vi "LVClass_WavefrontCorrectorSet Reset WavefrontCorrectorParameter to DefaultValue.vi"(0 "WavefrontCorrectorSet in":refnum<class "WavefrontCorrectorSet.lvclass">, 11 "error in (no error)":errorcluster) -> (4 "WavefrontCorrectorSet out":refnum<class "WavefrontCorrectorSet.lvclass">, 15 "error out":errorcluster)   [LabVIEW 2020, in "WavefrontCorrectorSet.lvclass"]
doc: "WavefrontCorrector parameter default value getter for parameter of type\nboolean.\n\n--------------------------------------------------------------------------------\n\n<B>wavefrontcorrector_setIn </B> : WavefrontCorrectorSet object.\n<B>wavefrontcorrector_setOut </B> : WavefrontCorrectorSet object.\n<B>parameter_name </B> : Parameter name.\n<B>default_value </B> : Parameter default value.\n<B>ErrorIn </B> : Error\n<B>ErrorOut </B> : Error\n\n--------------------------------------------------------------------------------"
uses:
  WavefrontCorrectorSet.lvclass
  WavefrontCorrectorSet.lvclass/WavefrontCorrectorSet.ctl
panel:
  in  "ListOfParametersToResetDefault":string[](array[string])
  in  "ResetAllParametersToDefault":bool
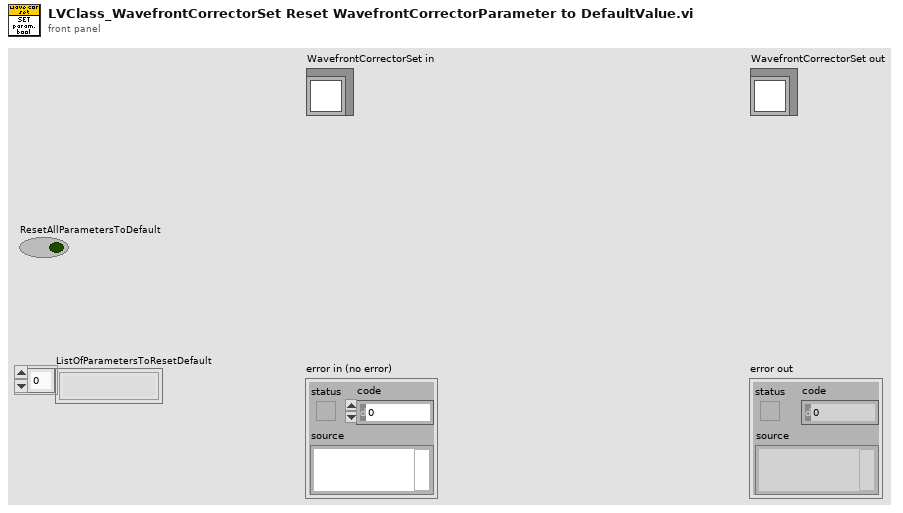
[diagram p1: front panel]
types:
  T1 = typedef "CameraParametersSetup.ctl" = cluster{"Name":string, "Type":T2, "Value":dbl, "BooleanValue":bool, "StringValue":string, "ConnectionParameter":bool}
  T2 = typedef "CameraParameters_Type.ctl" = enum16{"Integer", "Real", "String", "Boolean"}
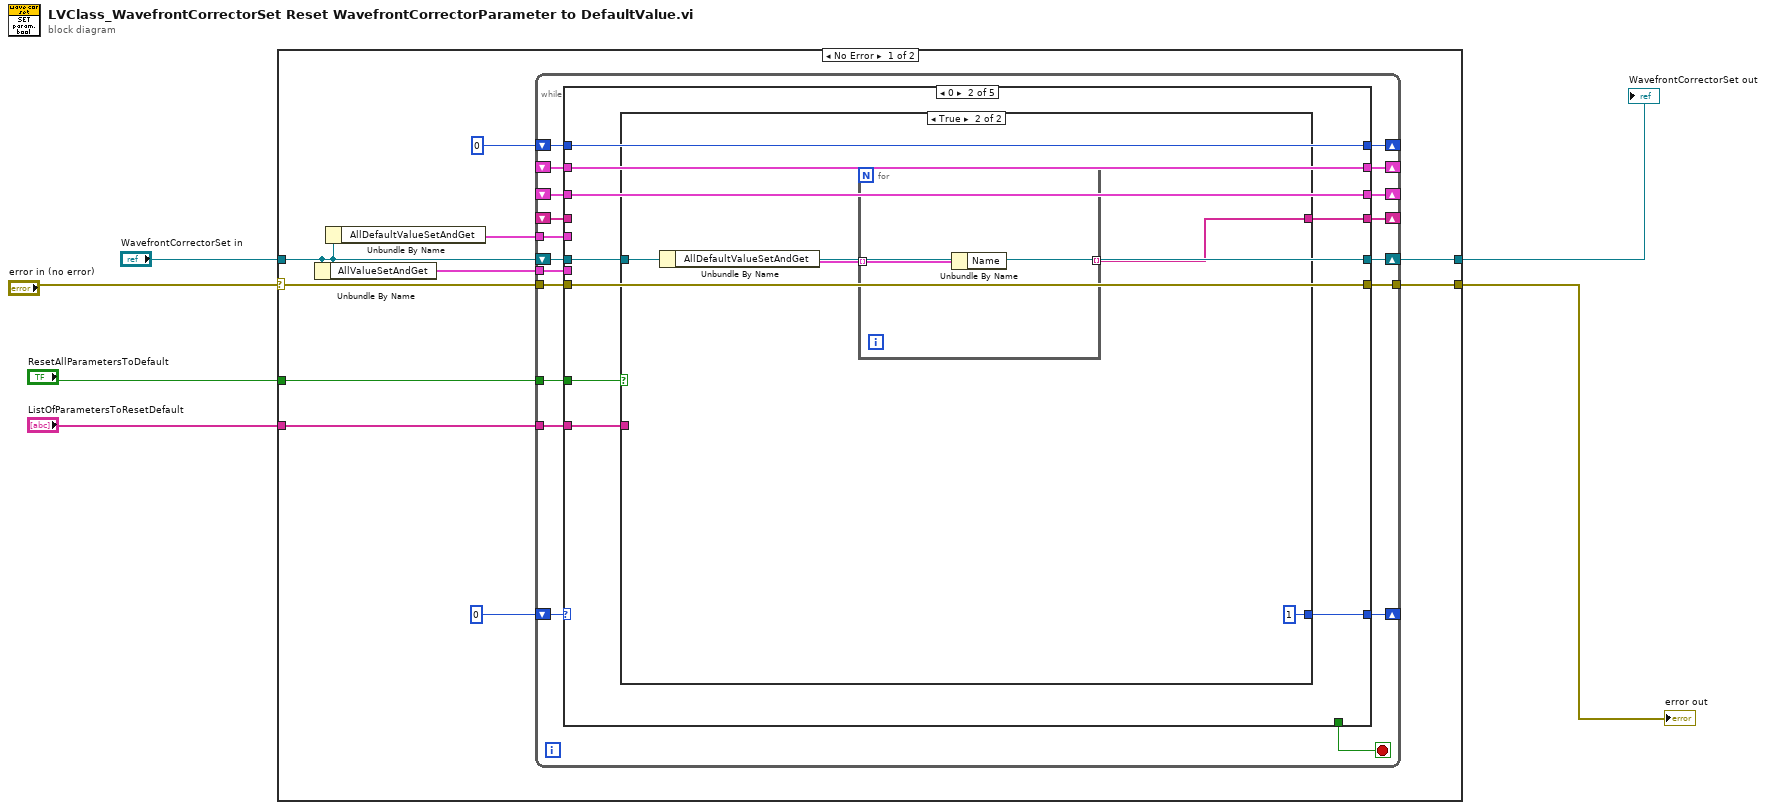
[diagram p0: block diagram]
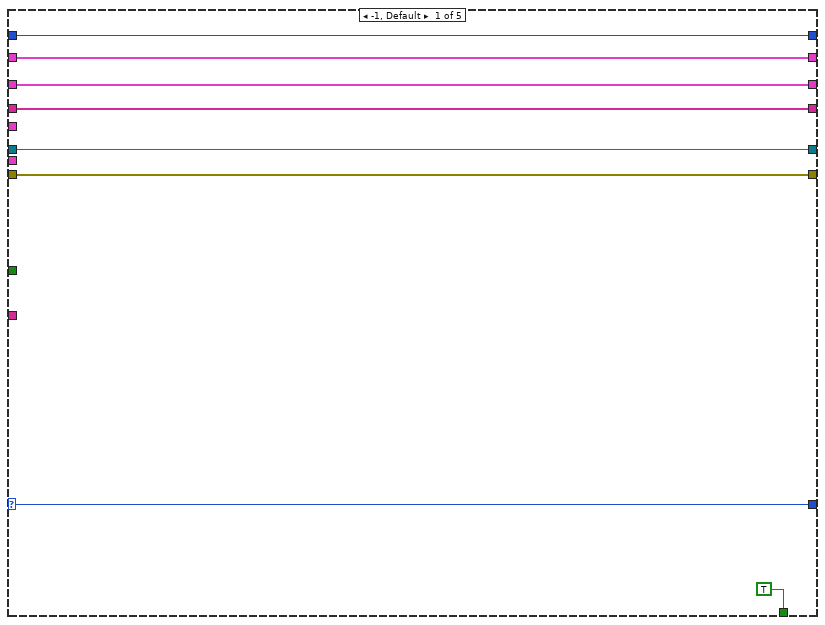
[diagram p2: hidden frame]
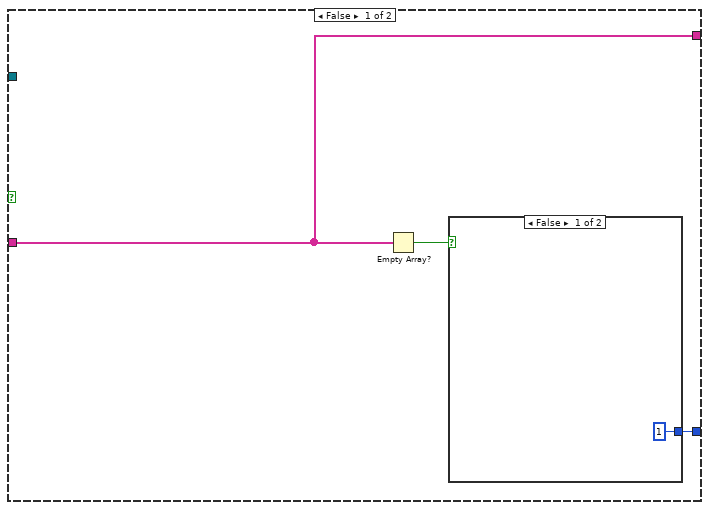
[diagram p3: hidden frame]
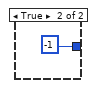
[diagram p4: hidden frame]
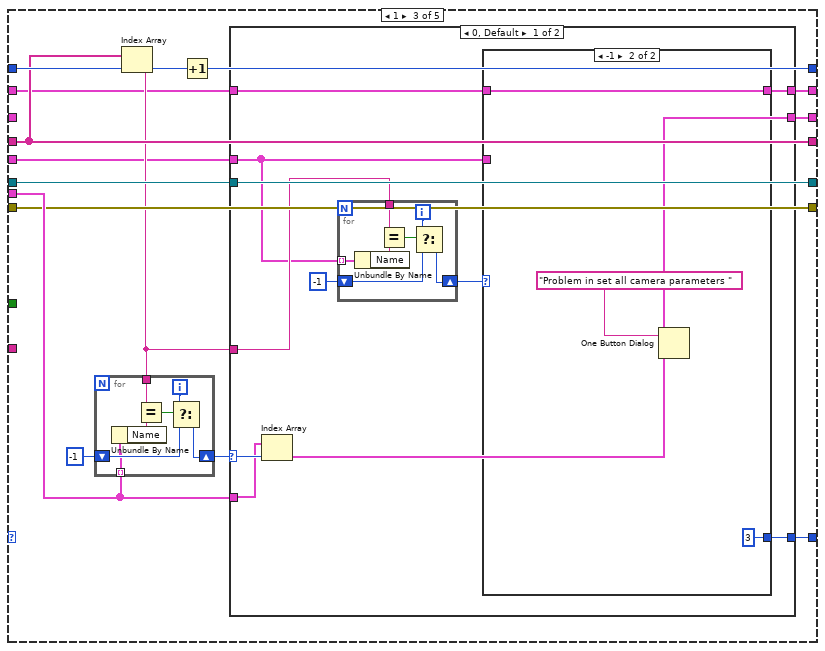
[diagram p5: hidden frame]
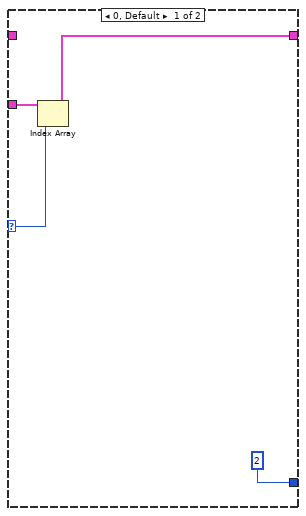
[diagram p6: hidden frame]
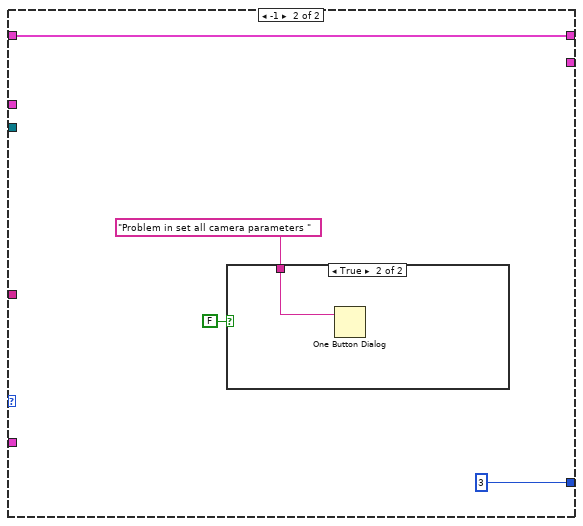
[diagram p7: hidden frame]
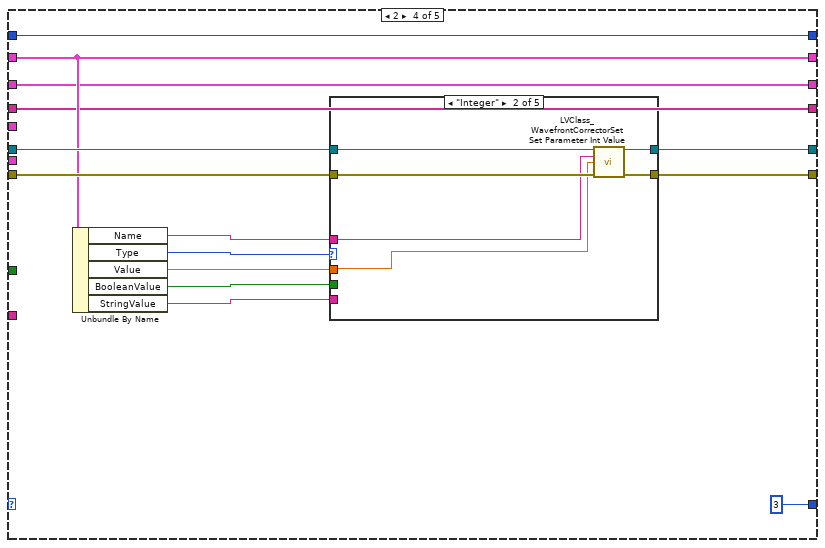
[diagram p9: hidden frame]
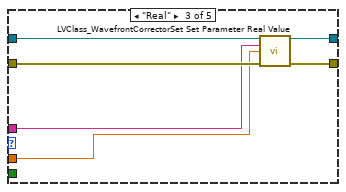
[diagram p11: hidden frame]
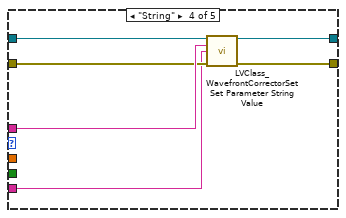
[diagram p12: hidden frame]
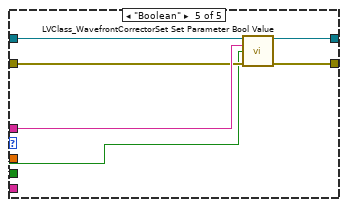
[diagram p13: hidden frame]
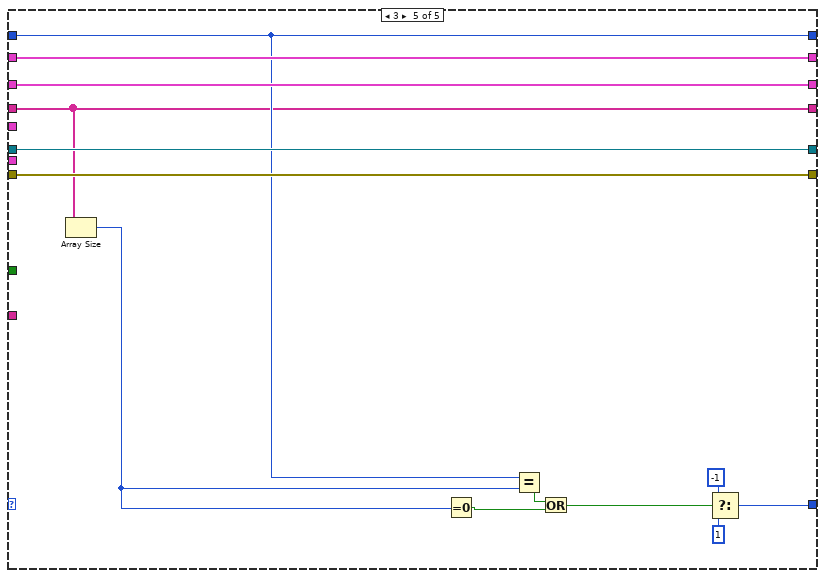
[diagram p14: hidden frame]
diagram:
  n1 = case shown="No Error" "error in (no error)" {
    selector: "error in (no error)" -> [w11 w168]
    tunnel: [w14 w168] -> w1
    tunnel: [w15 w167] -> w2
    tunnel: "WavefrontCorrectorSet in" -> [w10 w167]
    tunnel: "ResetAllParametersToDefault" -> [w8 _]
    tunnel: "ListOfParametersToResetDefault" -> [w7 _]
    frame No Error {
      n2 = Unbundle By Name(w10) -> ("AllValueSetAndGet"=w12:T1[])
      n3 = Unbundle By Name(w10) -> ("AllDefaultValueSetAndGet"=w9:T1[])
      n4 = while {
        tunnel: w11 -> [w31]
        shift-right: [w34] -> _
        shift-left: 0 -> [w35]
        tunnel: w12 -> [w29]
        tunnel: [w30] -> w14
        shift-right: [w32] -> w15
        shift-left: w10 -> [w33]
        shift-right: [w23] -> _
        shift-left: 0 -> [w26]
        shift-right: [w25] -> _
        shift-left: _ -> [w24]
        shift-right: [w22] -> _
        shift-left: _ -> [w21]
        shift-right: [w20] -> _
        shift-left: _ -> [w28]
        tunnel: w9 -> [w19]
        tunnel: w8 -> [w18]
        tunnel: w7 -> [w17]
        stop <- w27 stop-if-true
        n5 = case shown="0" w35 {
          selector: w35 -> [w37 _ _ _ _]
          tunnel: [w37 w44 w72 3 w161] -> w34
          tunnel: w33 -> [w43 w48 w71 w126 w164]
          tunnel: [w43 w48 w71 w125 w164] -> w32
          tunnel: w31 -> [w42 w47 w74 w124 w163]
          tunnel: [w42 w47 w74 w123 w163] -> w30
          tunnel: w29 -> [_ _ w77 _ _]
          tunnel: w28 -> [w36 _ w68 w114 w154]
          tunnel: [TRUE _ _ _ _] -> w27
          tunnel: w26 -> [w38 w51 w73 w116 w162]
          tunnel: [w40 w52 w65 w122 w166] -> w25
          tunnel: w24 -> [w40 w52 w64 w122 w166]
          tunnel: [w38 w51 w70 w116 w162] -> w23
          tunnel: [w39 w50 w69 w115 w165] -> w22
          tunnel: w21 -> [w39 w50 _ w115 w165]
          tunnel: [w36 w49 w68 w114 w154] -> w20
          tunnel: w19 -> [_ _ w66 _ _]
          tunnel: w18 -> [_ w46 _ _ _]
          tunnel: w17 -> [_ w45 _ _ _]
          frame -1, Default {
          }
          frame 0 {
            n6 = case shown="True" w46 {
              tunnel: [w55 w60] -> w49
              tunnel: w48 -> [_ w59]
              tunnel: w45 -> [w55 _]
              tunnel: [w54 1] -> w44
              frame False {
                n7 = Empty Array?(array=w55) -> (empty?=w53:bool)
                n8 = case shown="False" w53 {
                  tunnel: [1 -1] -> w54
                  frame False {
                  }
                  frame True {
                  }
                }
              }
              frame True {
                n9 = Unbundle By Name(w59) -> ("AllDefaultValueSetAndGet"=w61:T1[])
                n10 = for {
                  tunnel: w61 -> [w63] mode=indexing
                  tunnel: [w62] -> w60 mode=indexing
                  n11 = Unbundle By Name(w63) -> ("Name"=w62:string)
                }
              }
            }
          }
          frame 1 {
            n12 = Index Array(array=w68, index=w73) -> (element=w67:string)
            n13 = for {
              tunnel: w67 -> [w112]
              shift-right: [w109] -> w75
              shift-left: -1 -> [w108]
              tunnel: w77 -> [w107] mode=indexing
              i -> [w110]
              n14 = Unbundle By Name(w107) -> ("Name"=w113:string)
              n15 = Equal?(x=w112, y=w113) -> (x = y?=w111:bool)
              n16 = Select(t=w110, s=w111, f=w108) -> (s? t:f=w109:i32)
            }
            n17 = Increment(x=w73) -> (x+1=w70:i32)
            n18 = case shown="0, Default" w75 {
              selector: w75 -> [w87 _]
              tunnel: w77 -> [w86 _]
              tunnel: [w84 3] -> w72
              tunnel: w71 -> [_ _]
              tunnel: w67 -> [w82 _]
              tunnel: [w85 _] -> w69
              tunnel: w66 -> [w81 _]
              tunnel: [w80 w102] -> w65
              tunnel: w64 -> [w79 w102]
              frame 0, Default {
                n19 = Index Array(array=w86, index=w87) -> (element=w85:T1)
                n20 = for {
                  tunnel: w82 -> [w100]
                  shift-right: [w97] -> w78
                  shift-left: -1 -> [w96]
                  tunnel: w81 -> [w95] mode=indexing
                  i -> [w98]
                  n21 = Unbundle By Name(w95) -> ("Name"=w101:string)
                  n22 = Equal?(x=w100, y=w101) -> (x = y?=w99:bool)
                  n23 = Select(t=w98, s=w99, f=w96) -> (s? t:f=w97:i32)
                }
                n24 = case shown="-1" w78 {
                  selector: w78 -> [w88 _]
                  tunnel: [2 3] -> w84
                  tunnel: w81 -> [w90 _]
                  tunnel: [w89 w92] -> w80
                  tunnel: w79 -> [_ w92]
                  frame 0, Default {
                    n25 = Index Array(array=w90, index=w88) -> (element=w89:T1)
                  }
                  frame -1 {
                    n26 = One Button Dialog(message="Problem in set all camera parameters ") -> ()  [unwired: 1 in, 1 out]
                  }
                }
              }
              frame -1 {
                n27 = case shown="True" FALSE {
                  tunnel: "Problem in set all camera parameters " ("message") -> [_ w106]
                  frame False {
                  }
                  frame True {
                    n28 = One Button Dialog(message=w106) -> ()  [unwired: 1 in, 1 out]
                  }
                }
              }
            }
          }
          frame 2 {
            n29 = Unbundle By Name(w122) -> ("Name"=w117:string, "Type"=w121:T2, "Value"=w118:dbl, "BooleanValue"=w120:bool, "StringValue"=w119:string)
            n30 = case shown="\"Integer\"" w121 {
              tunnel: w117 -> [_ w130 w137 w146 w152]
              tunnel: w126 -> [w129 w135 w141 w147 w153]
              tunnel: [w129 w133 w139 w144 w150] -> w125
              tunnel: [w128 w132 w138 w143 w149] -> w123
              tunnel: w124 -> [w128 w134 w140 w145 w151]
              tunnel: w118 -> [_ w131 w136 _ _]
              tunnel: w120 -> [_ _ _ _ w148]
              tunnel: w119 -> [_ _ _ w142 _]
              frame Default {
              }
              frame "Integer" {
                n31 = call "LVClass_WavefrontCorrectorSet Set Parameter Int Value.vi"("WavefrontCorrectorSet in"=w135, "parameter_name"=w130, "Value"=w131, "error in (no error)"=w134) -> ("WavefrontCorrectorSet out"=w133:refnum<class "WavefrontCorrectorSet.lvclass">, "error out"=w132:errorcluster)  [unwired: 10 in]
              }
              frame "Real" {
                n32 = call "LVClass_WavefrontCorrectorSet Set Parameter Real Value.vi"("WavefrontCorrectorSet in"=w141, "parameter_name"=w137, "Value"=w136, "error in (no error)"=w140) -> ("WavefrontCorrectorSet out"=w139:refnum<class "WavefrontCorrectorSet.lvclass">, "error out"=w138:errorcluster)  [unwired: 10 in]
              }
              frame "String" {
                n33 = call "LVClass_WavefrontCorrectorSet Set Parameter String Value.vi"("WavefrontCorrectorSet in"=w147, "parameter name"=w146, "Value"=w142, "error in (no error)"=w145) -> ("WavefrontCorrectorSet out"=w144:refnum<class "WavefrontCorrectorSet.lvclass">, "error out"=w143:errorcluster)  [unwired: 10 in]
              }
              frame "Boolean" {
                n34 = call "LVClass_WavefrontCorrectorSet Set Parameter Bool Value.vi"("WavefrontCorrectorSet in"=w153, "parameter_name"=w152, "Value"=w148, "error in (no error)"=w151) -> ("WavefrontCorrectorSet out"=w150:refnum<class "WavefrontCorrectorSet.lvclass">, "error out"=w149:errorcluster)  [unwired: 10 in]
              }
            }
          }
          frame 3 {
            n35 = Array Size(array=w154) -> (size(s)=w155:i32)
            n36 = Equal To 0?(x=w155) -> (x = 0?=w158:bool)
            n37 = Equal?(x=w162, y=w155) -> (x = y?=w157:bool)
            n38 = Or(x=w157, y=w158) -> (x .or. y?=w156:bool)
            n39 = Select(t=-1, s=w156, f=1) -> (s? t:f=w161:i32)
          }
        }
      }
    }
    frame Error {
    }
  }
  "error out" <- w1
  "WavefrontCorrectorSet out" <- w2
